vi "Add-to-processing-buffer.vi"(6 "Index":i32, 7 "Time":timestamp, 8 "error in (no error)":errorcluster, 9 "Image ok?":bool, 10 "Images":T1[](array[typedef]), 11 "Buffers in":refnum<class "CV-Buffers.lvclass">) -> (0 "error out":errorcluster, 1 "Buffer ok?":bool, 3 "Buffers out":refnum<class "CV-Buffers.lvclass">)   [LabVIEW 2013, in "CameraVision.lvlib" / "CV-Main.lvclass"]
uses:
  CV-Main.lvclass
  Buffers/CV-Buffers.lvclass
  <vilib>/vision/Image Controls.llb/IMAQ Image.ctl
  Buffers/Processing-buffer.ctl
  Buffers/CV-Buffers.lvclass/CV-Buffers.ctl
  Buffers/Read Processing buffer.vi
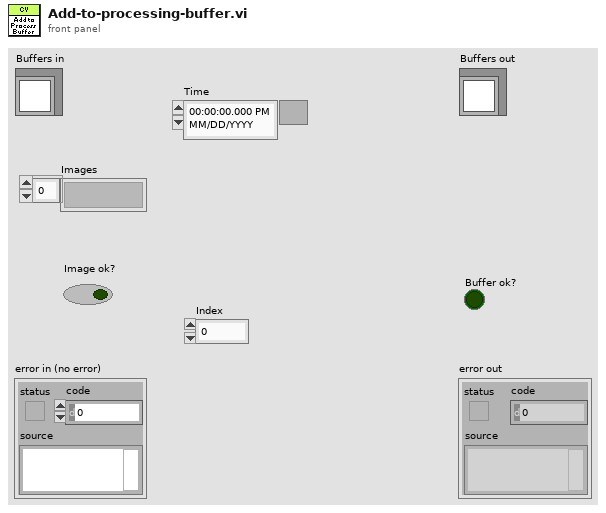
[diagram p1: front panel]
types:
  T1 = typedef "IMAQ Image.ctl" = refnum<image>
  T2 = typedef "CameraVision.lvlib/CV-Buffers.lvclass/Processing-buffer.ctl" = cluster{"Index":i32, "Time":timestamp, "Raw images":T1[]}
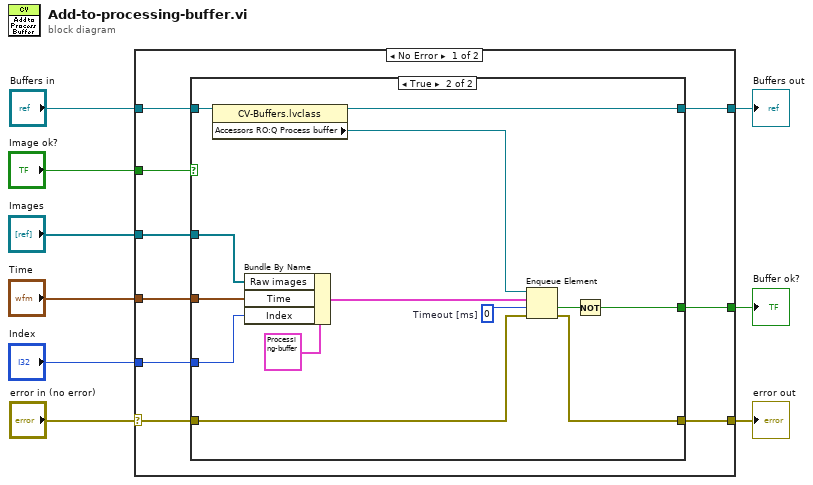
[diagram p0: block diagram]
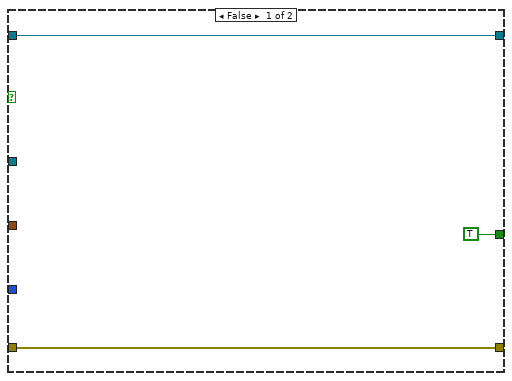
[diagram p2: hidden frame]
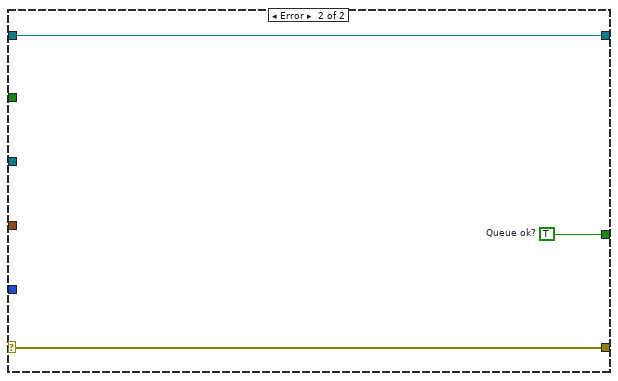
[diagram p3: hidden frame]
diagram:
  n1 = case shown="No Error" "error in (no error)" {
    selector: "error in (no error)" -> [w14 w37]
    tunnel: [w13 w37] -> w8
    tunnel: [w11 w36] -> w6
    tunnel: "Buffers in" -> [w18 w36]
    tunnel: "Images" -> [w17 _]
    tunnel: "Time" -> [w16 _]
    tunnel: "Index" -> [w15 _]
    tunnel: [w12 w35] -> w2
    tunnel: "Image ok?" -> [w10 _]
    frame No Error {
      n2 = case shown="True" w10 {
        tunnel: w18 -> [w21 w24]
        tunnel: w17 -> [_ w34]
        tunnel: w16 -> [_ w33]
        tunnel: w15 -> [_ w32]
        tunnel: w14 -> [w20 w28]
        tunnel: [w20 w27] -> w13
        tunnel: [TRUE w25] -> w12
        tunnel: [w21 w23] -> w11
        frame False {
        }
        frame True {
          w30 = 0  # Timeout [ms]
          n3 = property class="CV-Buffers.lvclass"(reference=w24) -> (reference out=w23:refnum<class "CV-Buffers.lvclass">, "Accessors RO:Q Process buffer"=w22:refnum<queue>)  [unwired: 1 in, 1 out]
          n4 = Bundle By Name(cluster=T2 {"Index"=0, "Time"=timestamp(0 s since 1904-01-01), "Raw images"=[]}, "Raw images"=w34, "Time"=w33, "Index"=w32) -> (w29:T2)
          n5 = Enqueue Element(queue=w22, element=w29, timeout in ms (-1)=w30, error in (no error)=w28) -> (timed out?=w26:bool, error out=w27:errorcluster)  [unwired: 1 out]
          n6 = Not(x=w26) -> (.not. x?=w25:bool)
        }
      }
    }
    frame Error {
      w35 = TRUE  # Queue ok?
    }
  }
  "error out" <- w8
  "Buffers out" <- w6
  "Buffer ok?" <- w2
